vi "group_XY.vi"(4 "Y_col":i32=2, 6 "X_col":i32=1, 7 "GroupBy_col":i32, 10 "data IN":dbl[][](array[numeric])) -> (2 "XY":cluster{"x_vals":dbl[], "y_vals":dbl[]}[](array[cluster]))   [LabVIEW 2013, in "tools.lvlib"]
uses:
  tools.lvlib
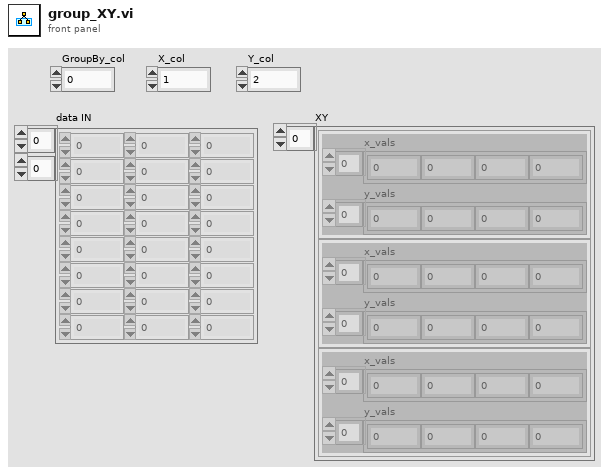
[diagram p1: front panel]
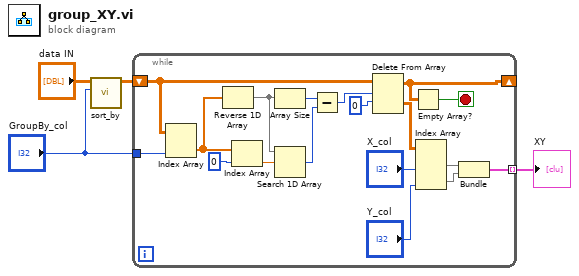
[diagram p0: block diagram]
diagram:
  n1 = call "sort_by.vi"("column index"="GroupBy_col", "data IN"="data IN") -> ("data OUT"=w3:dbl[][])  [unwired: 9 in]
  n2 = while {
    shift-right: [w20] -> _
    shift-left: w3 -> [w21]
    tunnel: "GroupBy_col" -> [w22]
    tunnel: [w5] -> w1 mode=indexing
    stop <- w19 stop-if-true
    n3 = Index Array(array=w21, index (col)=w22) -> (element=w17:dbl[])  [unwired: 1 in]
    n4 = Reverse 1D Array(array=w17) -> (reversed array=w15:dbl[])
    n5 = Index Array(array=w17, index=0) -> (element=w16:dbl)
    n6 = Array Size(array=w15) -> (size(s)=w13:i32)
    n7 = Search 1D Array(1D array=w15, element=w16) -> (index of element=w12:i32)  [unwired: 1 in]
    n8 = Subtract(x=w13, y=w12) -> (x-y=w14:i32)
    n9 = Delete From Array(array=w21, length=w14, index (row)=0) -> (deleted portion=w10:dbl[][], array with subset deleted=w20:dbl[][])  [unwired: 1 in]
    n10 = Empty Array?(array=w20) -> (empty?=w19:bool)
    n11 = Index Array(array=w10, index (col) #1="X_col", index (col) #2="Y_col") -> (element #1=w7:dbl[], element #2=w6:dbl[])  [unwired: 2 in]
    n12 = Bundle("data OUT"=w7, "data OUT"=w6) -> (w5:cluster{"data OUT":dbl[], "data OUT":dbl[]})  [unwired: 1 in]
  }
  "XY" <- w1
